vi "Configure.vi"(6 "Send Flow?":bool, 8 "error in (no error)":errorcluster, 9 "Analog_Configuration_Parameters":T1, 10 "Config Data":T2) -> (0 "error out":errorcluster, 3 "C100L out":refnum<class "C100L.lvclass">)   [LabVIEW 2021, in "C100L.lvlib" / "C100L.lvclass"]
uses:
  C100L.lvclass
  C100L.lvclass/C100L.ctl
  Config Data.ctl
  <vilib>/NathanCo/Analog-Tasks/Utilities/Analog Configuration Parameters.ctl
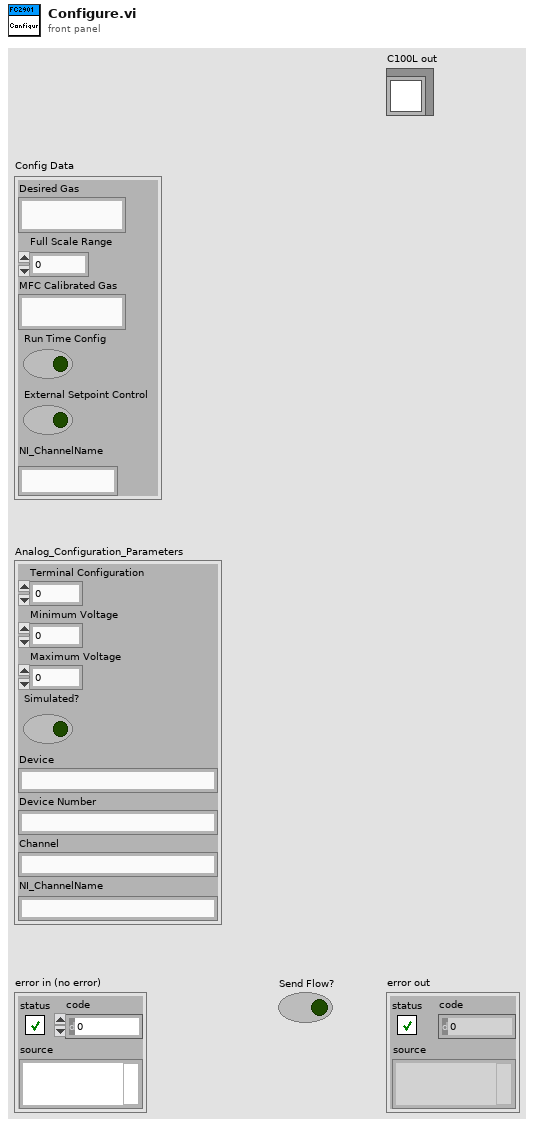
[diagram p1: front panel]
types:
  T1 = typedef "Analog Configuration Parameters.ctl" = cluster{"Terminal Configuration":i32, "Minimum Voltage":dbl, "Maximum Voltage":dbl, "Simulated?":bool, "Device":string, "Device Number":string, "Channel":string, "NI_ChannelName":string}
  T2 = typedef "C100L.lvlib/C100L.lvclass/Config Data.ctl" = cluster{"Desired Gas":string, "Full Scale Range":dbl, "MFC Calibrated Gas":string, "Run Time Config":bool, "External Setpoint Control":bool, "NI_ChannelName":string}
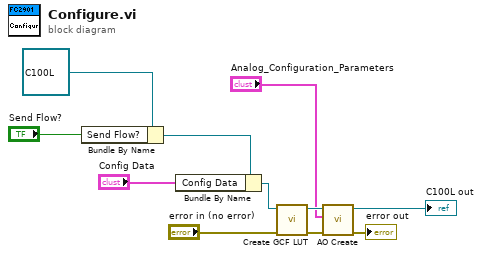
[diagram p0: block diagram]
diagram:
  n1 = Bundle By Name(cluster=refnum<class "C100L.lvclass"> refnum ("C100L.lvlib:C100L.lvclass"), "Send Flow?"="Send Flow?") -> (w4:refnum<class "C100L.lvclass">)
  n2 = Bundle By Name(cluster=w4, "Config Data"="Config Data") -> (w9:refnum<class "C100L.lvclass">)
  n3 = call "Create GCF LUT.vi"("error in (no error)"="error in (no error)", "C100L in"=w9) -> ("error out"=w5:errorcluster, "C100L out"=w7:refnum<class "C100L.lvclass">)  [unwired: 8 in]
  n4 = call "AO Create.vi"("error in (no error)"=w5, "Analog_Configuration_Parameters"="Analog_Configuration_Parameters", "C100L in"=w7) -> ("error out"=→"error out":errorcluster, "C100L out"=→"C100L out":refnum<class "C100L.lvclass">)  [unwired: 7 in]
